vi "bt_host.vi"() -> ()   [LabVIEW 2023]
uses:
  <vilib>/Platform/TimedLoop/XDataNode/timing_clust.ctl
  <vilib>/Platform/TimedLoop/XDataNode/nitl_modes.ctl
  <vilib>/Platform/TimedLoop/XDataNode/wakeup.ctl
  <vilib>/Instr/_visa.llb/VISA Configure Serial Port (Instr).vi
  <vilib>/Platform/TimedLoop/XDataNode/XDataNode.xnode
  <vilib>/Platform/TimedLoop/XDataNode/XDNodeRunTimeDep.lvlib
panel:
  in  "탭 컨트롤 3":enum32{"Setting", "Main"}(tab)
  out "Gen ok?":bool
  out "Save_Name ok?":bool
  out "Data_Save_Name":i32[](array[numeric])
  in  "Packet Size":i32=60
  in  "설정 완료":bool
  in  "VISA resource":refnum<visa-resource-name>="COM3"
  in  "Gender":enum32{"Male", "Female"}(radio)
  in  "age":dbl
  in  "height":dbl
  out "Jitter":i32
  out "Total Data Len":i32
  out "Data":i32[](array[numeric])
  out "Received Message Count":i32
  out "Dataset":i32[](array[numeric])
  out "Adaptability(%)":sgl format="%#_3g"
  out "Batt":sgl format="%#_3g"
  in  "탭 컨트롤 2":enum32{"R/L Control", "Total Control"}(tab)
  in  "R Set":bool
  in  "R_Peak Force":i32
  in  "R_Peak":i32
  in  "R_Onset":i32
  in  "R_Release":i32
  in  "L_Release":i32
  in  "L_Onset":i32
  in  "L_Peak":i32
  in  "L_Peak Force":i32
  in  "L_Set":bool
  in  "T_Set":bool
  in  "T_Peak Force":i32
  in  "T_Peak":i32
  in  "T_Onset":i32
  in  "T_Release":i32
  in  "System Stop":bool
  in  "Stop":bool
  in  "start":bool
  out "R_GCP(%)":sgl(slide) scale=0.0..100.0
  out "L_GCP(%)":sgl(slide) scale=0.0..100.0
  in  "Control Main On/Off":bool
  out "Gait Value":cluster{"[0]":sgl, "[1]":sgl}(graph)
  out "Force":T1(graph)
  out "IMU Deg":cluster{"[0]":sgl, "[1]":sgl}(graph)
  out "COM Port":refnum<visa-resource-name>
  # "Batt(%)"
  # "Right Force Control"
  # "Left Force Control"
  # "Total Force Control"
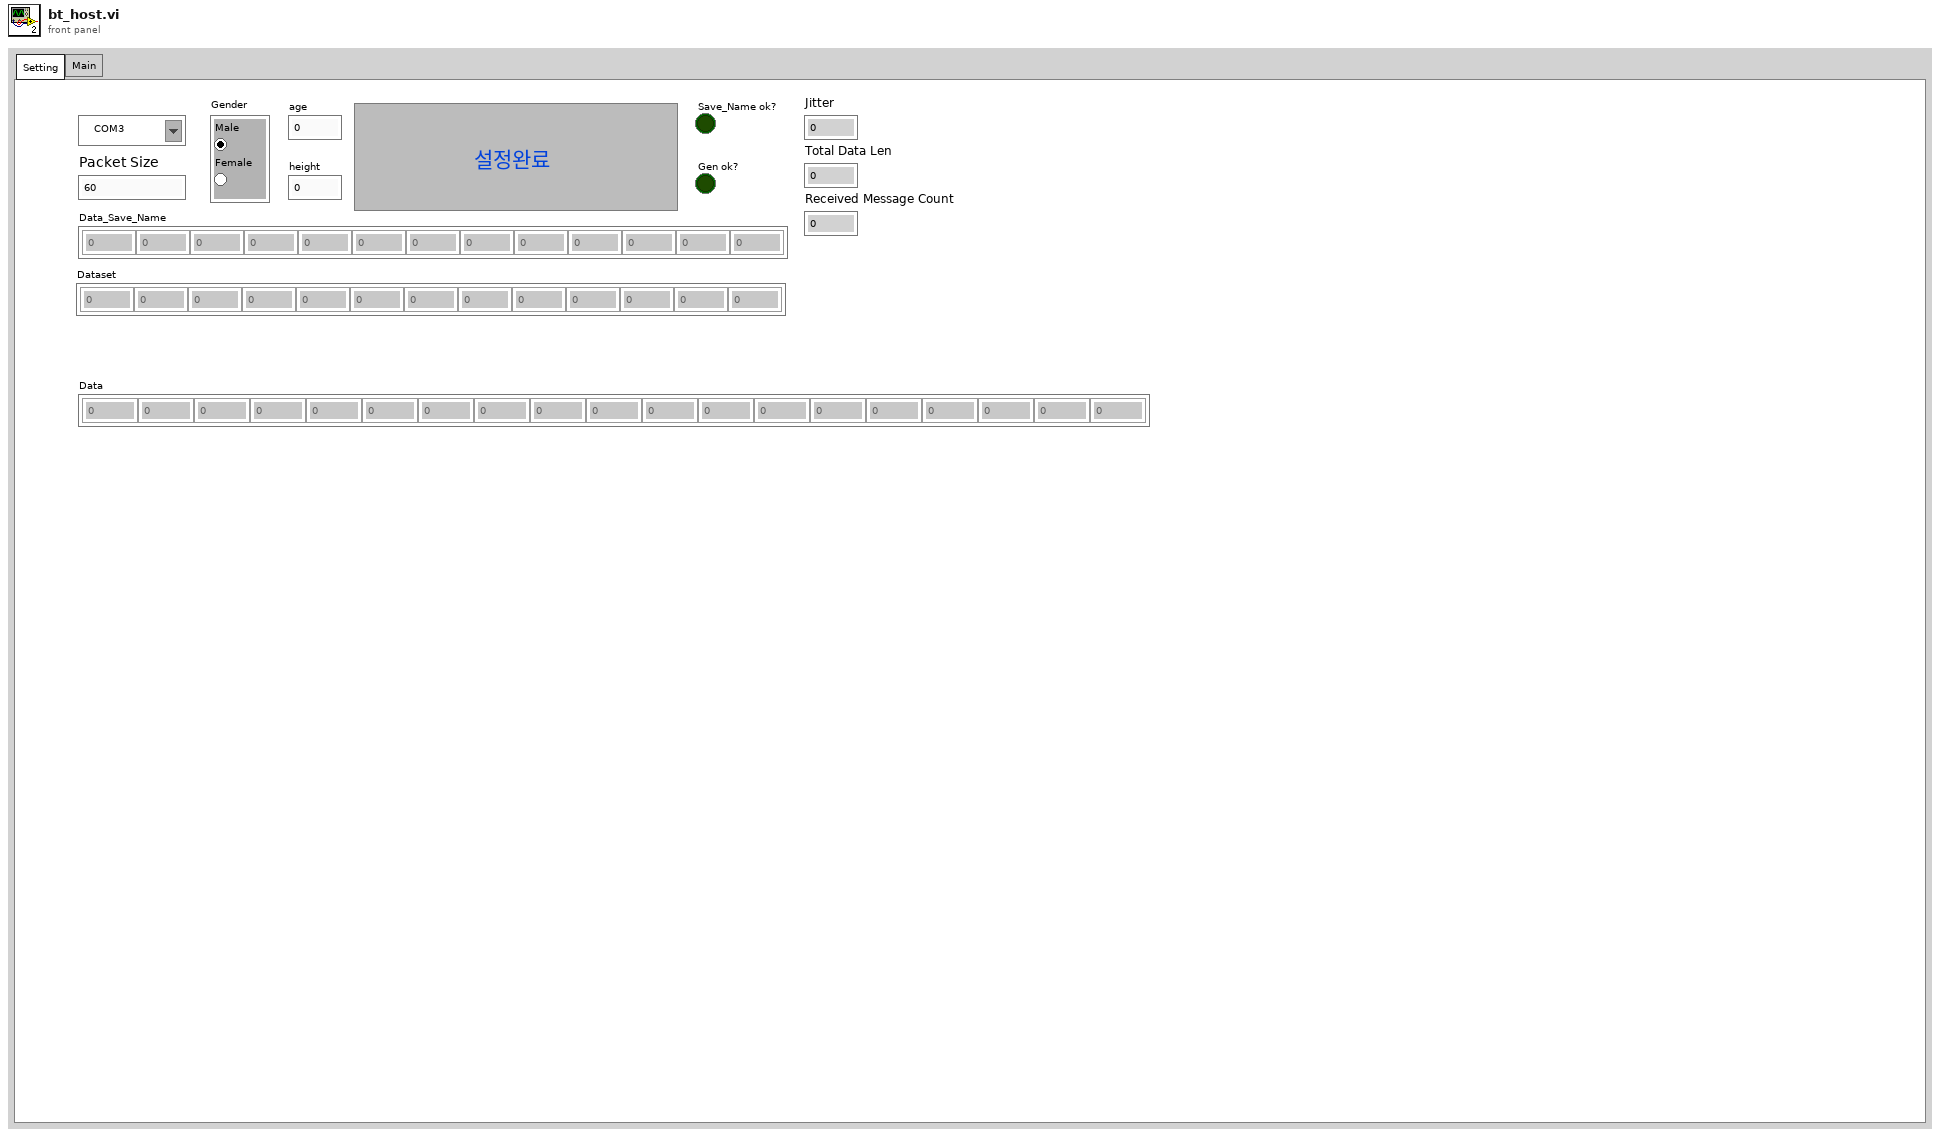
[diagram p1: front panel]
types:
  T1 = cluster{"[0]":sgl, "[1]":sgl, "[2]":sgl, "[3]":sgl}
  T2 = typedef "XDNodeRunTimeDep.lvlib/timing_clust.ctl" = cluster{"Expected End [f-1]":u64, "Actual End [f-1]":u64, "Finished Late? [f-1]":bool, "Expected End [i-1]":u64, "Actual End [i-1]":u64, "Finished Late? [i-1]":bool, "Expected Start [i]":u64, "Actual Start [i]":u64, "Expected Start [f]":u64, "Actual Start [f]":u64, "Source Name":string, "Structure Name":string, "Period":i64, "Deadline":i64, "Offset":i64, "Start":i64, "Priority":i32, "Timeout":i32, "Mode":T3, "Wakeup Reason":T4, "Error":errorcluster, "Source Type":string, "Secondary Source Type":string, "Global End Time":u64, "Global Start Time":u64, "Frame Duration":u64, "Iteration Duration":u64, "Assigned CPU":i32, "I/O Scan Engine Mode":u32}
  T3 = typedef "XDNodeRunTimeDep.lvlib/nitl_modes.ctl" = enum32{"No Change", "Process missed periods, maintain original phase", "Discard missed periods, maintain original phase", "Process missed periods, ignore original phase", "Discard missed periods, ignore original phase"}
  T4 = typedef "XDNodeRunTimeDep.lvlib/wakeup.ctl" = enum32{"Normal", "Aborted", "Asynchronous wakeup", "Timing source error", "Timed loop error", "Timeout"}
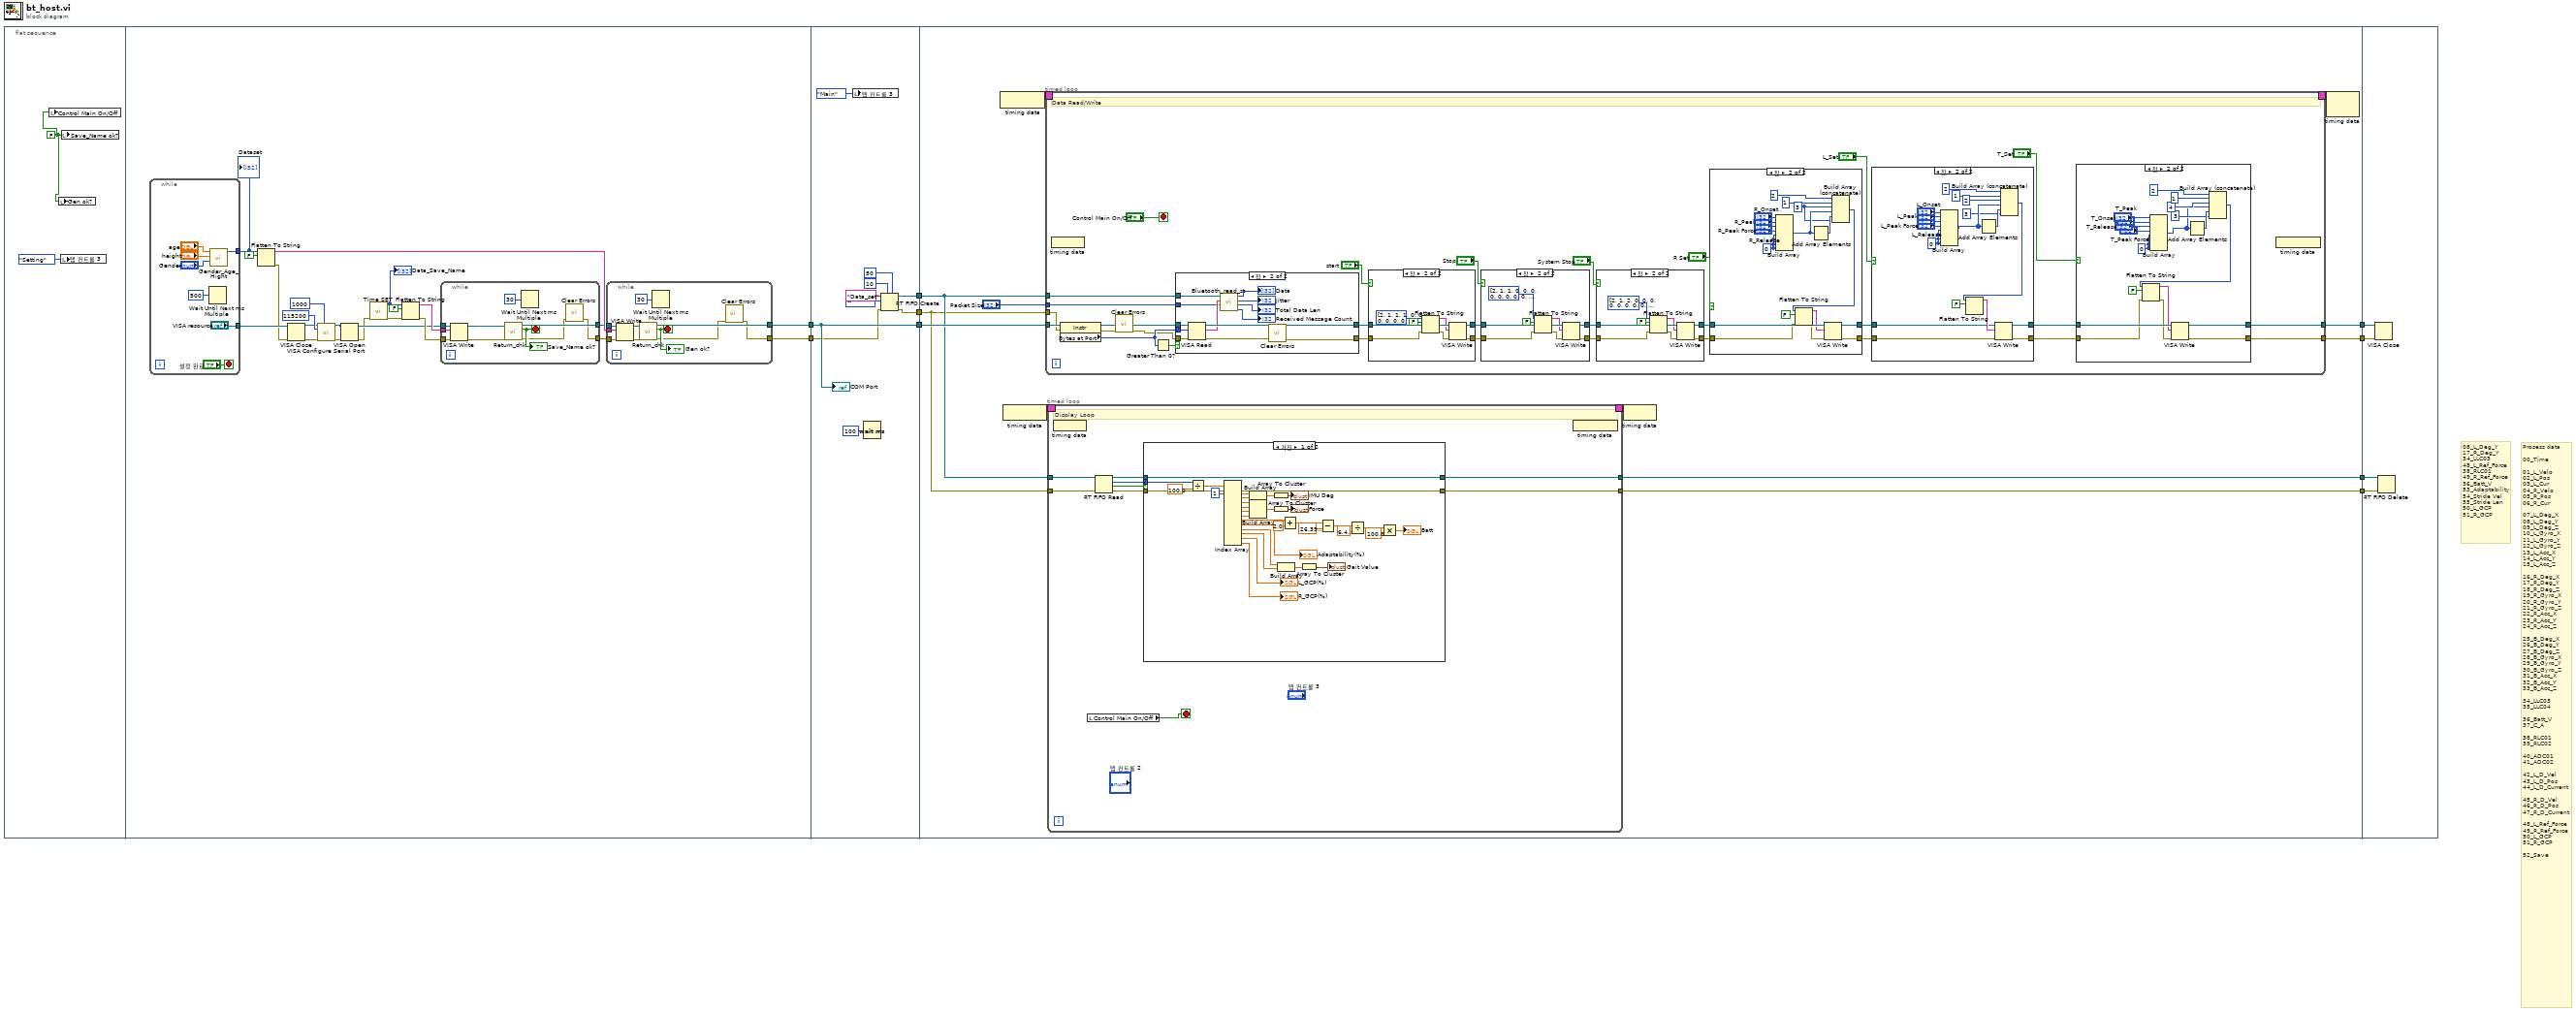
[diagram p0: block diagram]
diagram:
  # "08_L_Deg_Y\n17_R_Deg_Y\n34_LLC03\n48_L_Ref_Force\n38_RLC01\n49_R_Ref_Force\n36_Batt_V\n53_Adaptability\n54_Stride Vel\n55_Stride Len\n50_L_GCP\n51_R_GCP"
  # "Prosess data\n\n00_Time\n\n01_L_Velo\n02_L_Pos\n03_L_Cur\n04_R_Velo\n05_R_Pos\n06_R_Cur\n\n07_L_Deg_X\n08_L_Deg_Y\n09_L_Deg_Z\n10_L_Gyro_X\n11_L_Gyro_Y\n12_L_Gyro_Z\n13_L_Acc_X\n14_L_Acc_Y\n15_L_Acc_Z\n\n16_R_Deg_X\n17_R_Deg_Y\n18_R_Deg_Z\n19_R_Gyro_X\n20_R_Gyro_Y\n21_R_Gyro_Z\n22_R_Acc_X\n23_R_Acc_Y\n24_R_Acc_Z\n\n25_B_Deg_X\n26_B_Deg_Y\n27_B_Deg_Z\n28_B_Gyro_X\n29_B_Gyro_Y\n30_B_Gyro_Z\n31_B_Acc_X\n32_B_Acc_Y\n33_B_Acc_Z\n\n34_LLC03\n35_LLC04\n\n36_Batt_V\n37_C_A\n\n38_RLC01\n39_RLC02\n\n40_ADC01\n41_ADC02\n\n42_L_D_Vel\n43_L_D_Pos\n44_L_D_Current\n\n45_R_D_Vel\n46_R_D_Pos\n47_R_D_Current\n\n48_L_Ref_Force\n49_R_Ref_Force\n50_L_GCP\n51_R_GCP\n\n52_Save"
  n1 = flat-sequence {
    tunnel: [w15] -> w9
    tunnel: [w14] -> w7
    tunnel: w9 -> [w69]
    tunnel: [w69] -> w8
    tunnel: w7 -> [w66]
    tunnel: [w63] -> w6
    tunnel: [w61] -> w1
    tunnel: w8 -> [w81]
    tunnel: w6 -> [w73]
    tunnel: [w77] -> w5
    tunnel: [w76] -> w4
    tunnel: [w72] -> w3
    tunnel: [w71] -> w2
    tunnel: w1 -> [w70]
    tunnel: w5 -> [w272]
    tunnel: w4 -> [w271]
    tunnel: w3 -> [w270]
    tunnel: w2 -> [w269]
    frame #0 {
      w11 = FALSE ("Save_Name ok?")
      n2 = local write "Control Main On/Off"(w11) -> ()
      n3 = local write "Gen ok?"(w11) -> ()
      n4 = local write "탭 컨트롤 3"(enum32{"Setting", "Main"}."Setting" ("탭 컨트롤 3")) -> ()
      n5 = local write "Save_Name ok?"(w11) -> ()
    }
    frame #1 {
      n6 = while {
        tunnel: ["VISA resource"] -> w28
        tunnel: [w53] -> w18
        stop <- "설정 완료" stop-if-true
        n7 = Wait Until Next ms Multiple(millisecond multiple=u32 500 ("ms 배수")) -> ()  [unwired: 1 out]
        n8 = call "Gender_Age_Hight.vi"("Gender"="Gender", "height"="height", "age"="age") -> ("Dataset"=w53:i32[])  [unwired: 8 in]
      }
      "Dataset" <- w18
      n9 = Flatten To String(anything=w18, prepend array or string size? (T)=FALSE ("배열 또는 문자열 크기를 앞에 추가? (참)")) -> (data string=w17:string, error out=w16:errorcluster)  [unwired: 2 in, 1 out]
      n10 = VISA Close(VISA resource name=w28, error in (no error)=w16) -> (error out=w27:errorcluster)
      n11 = call-poly "VISA Configure Serial Port"("VISA resource name"=w28, "timeout (10sec)"=u32 1000, "baud rate (9600)"=u32 115200, "error in (no error)"=w27) -> ("VISA resource name out"=w30:refnum<visa-resource-name>, "error out"=w29:errorcluster)  [unwired: 10 in]
      n12 = VISA Open(error in (no error)=w29, VISA resource name=w30) -> (VISA resource name=w22:refnum<visa-resource-name>, error out=w20:errorcluster)  [unwired: 3 in]
      n13 = call "Time SET.vi"("Err_IN"=w20) -> ("Err_Out"=w21:errorcluster, "배열"=w25:i32[])  [unwired: 9 in]
      "Data_Save_Name" <- w25
      n14 = Flatten To String(anything=w25, prepend array or string size? (T)=FALSE ("배열 또는 문자열 크기를 앞에 추가? (참)"), error in (no error)=w21) -> (data string=w23:string, error out=w24:errorcluster)  [unwired: 1 in, 1 out]
      n15 = while {
        tunnel: w24 -> [w52]
        tunnel: w23 -> [w51]
        tunnel: w22 -> [w50]
        tunnel: [w43] -> w13
        tunnel: [w46] -> w12
        stop <- w47 stop-if-true
        n16 = VISA Write(VISA resource name=w50, write buffer=w51, error in (no error)=w52) -> (VISA resource name out=w49:refnum<visa-resource-name>, error out=w48:errorcluster)  [unwired: 1 out]
        n17 = call "Return_chk.vi"("에러 입력(에러 없음)"=w48, "VISA 참조 번호 입력"=w49) -> ("에러 출력"=w44:errorcluster, "불리언"=w47:bool, "VISA 참조 번호 출력"=w46:refnum<visa-resource-name>)  [unwired: 7 in]
        "Save_Name ok?" <- w47
        n18 = Wait Until Next ms Multiple(millisecond multiple=u32 30 ("ms 배수")) -> ()  [unwired: 1 out]
        n19 = call <vilib>:"Clear Errors.vi"("error in (no error)"=w44) -> ("error out"=w43:errorcluster)  [unwired: 5 in, 1 out]
      }
      n20 = while {
        tunnel: w13 -> [w42]
        tunnel: w17 -> [w41]
        tunnel: w12 -> [w40]
        tunnel: [w33] -> w14
        tunnel: [w36] -> w15
        stop <- w37 stop-if-true
        n21 = VISA Write(VISA resource name=w40, write buffer=w41, error in (no error)=w42) -> (VISA resource name out=w39:refnum<visa-resource-name>, error out=w38:errorcluster)  [unwired: 1 out]
        n22 = call "Return_chk.vi"("에러 입력(에러 없음)"=w38, "VISA 참조 번호 입력"=w39) -> ("에러 출력"=w34:errorcluster, "불리언"=w37:bool, "VISA 참조 번호 출력"=w36:refnum<visa-resource-name>)  [unwired: 7 in]
        "Gen ok?" <- w37
        n23 = Wait Until Next ms Multiple(millisecond multiple=u32 30 ("ms 배수")) -> ()  [unwired: 1 out]
        n24 = call <vilib>:"Clear Errors.vi"("error in (no error)"=w34) -> ("error out"=w33:errorcluster)  [unwired: 5 in, 1 out]
      }
    }
    frame #2 {
      n25 = local write "탭 컨트롤 3"(enum32{"Setting", "Main"}."Main" ("탭 컨트롤 3")) -> ()
      n26 = Wait (ms)(milliseconds to wait=u32 100 ("대기 시간 (ms)")) -> ()  [unwired: 1 out]
      n27 = RT FIFO Create(0:"Data_set" ("이름(이름없음)"), 1:i32[] [], 3:w66, 4:u32 10 ("크기(10)"), 6:u32 50 ("배열의 원소(1)")) -> (8:w63:refnum<k33>, 11:w61:errorcluster)  [unwired: 3 in, 1 out]
      "COM Port" <- w69
    }
    frame #3 {
      n28 = node-c288() -> (w80:T2)
      n29 = node-c288() -> (w75:T2)
      n30 = timed-loop {
        timing: w80 -> [_]
        timing-out: [_] -> w79
        tunnel: w81 -> [w158]
        tunnel: [w130] -> w76
        tunnel: [w129] -> w77
        tunnel: "Packet Size" -> [w154]
        tunnel: w73 -> [w153]
        tunnel: w70 -> [w152]
        stop <- "Control Main On/Off" stop-if-true
        # "Data Read/Write"
        n31 = node-c288() -> ()  [unwired: 1 in]
        n32 = property class="Instr"(reference=w158, error in=w152) -> (reference out=w156:refnum<visa-resource-name>, error out=w142:errorcluster, "Bytes at Port"=w155:u32)
        n33 = call <vilib>:"Clear Errors.vi"("error in (no error)"=w142) -> ("error out"=w141:errorcluster)  [unwired: 5 in, 1 out]
        n34 = Greater Than 0?(x=w155) -> (x > 0?=w157:bool)
        n35 = case shown="참" w157 {
          tunnel: w141 -> [w250 w263]
          tunnel: w156 -> [w251 w264]
          tunnel: w155 -> [_ w262]
          tunnel: [w251 w261] -> w150
          tunnel: [w250 w252] -> w149
          tunnel: w154 -> [_ w255]
          tunnel: w153 -> [_ w257]
          frame False {
          }
          frame True {
            n36 = VISA Read(VISA resource name=w264, byte count=w262, error in (no error)=w263) -> (VISA resource name out=w261:refnum<visa-resource-name>, read buffer=w256:string, error out=w253:errorcluster)  [unwired: 1 out]
            n37 = call "Bluetooth_read_st.vi"("Packet Size"=w255, "read buffer"=w256, "Data_set"=w257) -> ("Received Message Count"=→"Received Message Count":i32, "Total Data Len"=→"Total Data Len":i32, "Jitter"=→"Jitter":i32, "Data"=→"Data":i32[])  [unwired: 5 in]
            n38 = call <vilib>:"Clear Errors.vi"("error in (no error)"=w253) -> ("error out"=w252:errorcluster)  [unwired: 5 in, 1 out]
          }
        }
        n39 = case shown="참" "start" {
          tunnel: w150 -> [w241 w249]
          tunnel: w149 -> [w240 w244]
          tunnel: [w241 w248] -> w148
          tunnel: [w240 w247] -> w147
          frame False {
          }
          frame True {
            n40 = Flatten To String(anything=i32[] [2, 1, 1, 1, 0, 0, 0, 0, 0, 0, 0, 1, 3], prepend array or string size? (T)=FALSE ("배열 또는 문자열 크기를 앞에 추가? (참)"), error in (no error)=w244) -> (data string=w242:string, error out=w245:errorcluster)  [unwired: 1 in, 1 out]
            n41 = VISA Write(VISA resource name=w249, write buffer=w242, error in (no error)=w245) -> (VISA resource name out=w248:refnum<visa-resource-name>, error out=w247:errorcluster)  [unwired: 1 out]
          }
        }
        n42 = case shown="참" "Stop" {
          tunnel: w148 -> [w231 w239]
          tunnel: w147 -> [w230 w234]
          tunnel: [w231 w238] -> w145
          tunnel: [w230 w237] -> w144
          frame False {
          }
          frame True {
            n43 = Flatten To String(anything=i32[] [2, 1, 1, 0, 0, 0, 0, 0, 0, 0, 0, 0, 3], prepend array or string size? (T)=FALSE ("배열 또는 문자열 크기를 앞에 추가? (참)"), error in (no error)=w234) -> (data string=w233:string, error out=w235:errorcluster)  [unwired: 1 in, 1 out]
            n44 = VISA Write(VISA resource name=w239, write buffer=w233, error in (no error)=w235) -> (VISA resource name out=w238:refnum<visa-resource-name>, error out=w237:errorcluster)  [unwired: 1 out]
          }
        }
        n45 = case shown="참" "System Stop" {
          tunnel: w145 -> [w221 w229]
          tunnel: w144 -> [w220 w224]
          tunnel: [w221 w228] -> w140
          tunnel: [w220 w227] -> w139
          frame False {
          }
          frame True {
            n46 = Flatten To String(anything=i32[] [2, 1, 2, 0, 0, 0, 0, 0, 0, 0, 0, 2, 3], prepend array or string size? (T)=FALSE ("배열 또는 문자열 크기를 앞에 추가? (참)"), error in (no error)=w224) -> (data string=w223:string, error out=w225:errorcluster)  [unwired: 1 in, 1 out]
            n47 = VISA Write(VISA resource name=w229, write buffer=w223, error in (no error)=w225) -> (VISA resource name out=w228:refnum<visa-resource-name>, error out=w227:errorcluster)  [unwired: 1 out]
          }
        }
        n48 = case shown="참" "R Set" {
          tunnel: w140 -> [w201 w217]
          tunnel: w139 -> [w200 w214]
          tunnel: [w201 w219] -> w135
          tunnel: [w200 w218] -> w134
          frame False {
          }
          frame True {
            w206 = 0 ("원소")
            w203 = 3 ("원소")
            n49 = Build Array("R_Onset", "R_Peak", "R_Release", "R_Peak Force", w206, w206, w206, w206) -> (w205:i32[])
            n50 = Add Array Elements(numeric array=w205) -> (sum=w204:i32)
            n51 = Build Array (concatenate)(2 ("원소"), 1 ("원소"), w203, w205, w204, w203) -> (w202:i32[])
            n52 = Flatten To String(anything=w202, prepend array or string size? (T)=FALSE ("배열 또는 문자열 크기를 앞에 추가? (참)"), error in (no error)=w214) -> (data string=w216:string, error out=w215:errorcluster)  [unwired: 1 in, 1 out]
            n53 = VISA Write(VISA resource name=w217, write buffer=w216, error in (no error)=w215) -> (VISA resource name out=w219:refnum<visa-resource-name>, error out=w218:errorcluster)  [unwired: 1 out]
          }
        }
        n54 = case shown="참" "L_Set" {
          tunnel: w135 -> [w181 w193]
          tunnel: w134 -> [w180 w192]
          tunnel: [w180 w191] -> w132
          tunnel: [w181 w190] -> w133
          frame False {
          }
          frame True {
            w182 = 0 ("원소")
            n55 = Build Array("L_Onset", "L_Peak", "L_Release", "L_Peak Force", w182, w182, w182, w182) -> (w185:i32[])
            n56 = Add Array Elements(numeric array=w185) -> (sum=w187:i32)
            n57 = Build Array (concatenate)(2 ("원소"), 1 ("원소"), 2 ("원소"), w185, w187, 3 ("원소")) -> (w183:i32[])
            n58 = Flatten To String(anything=w183, prepend array or string size? (T)=FALSE ("배열 또는 문자열 크기를 앞에 추가? (참)")) -> (data string=w195:string)  [unwired: 2 in, 2 out]
            n59 = VISA Write(VISA resource name=w193, write buffer=w195, error in (no error)=w192) -> (VISA resource name out=w190:refnum<visa-resource-name>, error out=w191:errorcluster)  [unwired: 1 out]
          }
        }
        n60 = case shown="참" "T_Set" {
          tunnel: w133 -> [w160 w177]
          tunnel: w132 -> [w159 w174]
          tunnel: [w160 w179] -> w130
          tunnel: [w159 w178] -> w129
          frame False {
          }
          frame True {
            w172 = 0 ("원소")
            n61 = Build Array("T_Onset", "T_Peak", "T_Release", "T_Peak Force", w172, w172, w172, w172) -> (w162:i32[])
            n62 = Add Array Elements(numeric array=w162) -> (sum=w165:i32)
            n63 = Build Array (concatenate)(2 ("원소"), 1 ("원소"), 4 ("원소"), w162, w165, 3 ("원소")) -> (w161:i32[])
            n64 = Flatten To String(anything=w161, prepend array or string size? (T)=FALSE ("배열 또는 문자열 크기를 앞에 추가? (참)"), error in (no error)=w174) -> (data string=w175:string, error out=w176:errorcluster)  [unwired: 1 in, 1 out]
            n65 = VISA Write(VISA resource name=w177, write buffer=w175, error in (no error)=w176) -> (VISA resource name out=w179:refnum<visa-resource-name>, error out=w178:errorcluster)  [unwired: 1 out]
          }
        }
        n66 = node-c288() -> ()  [unwired: 1 out]
      }
      n67 = timed-loop {
        timing: w75 -> [_]
        timing-out: [_] -> w74
        tunnel: w73 -> [w90]
        tunnel: [w85] -> w71
        tunnel: [w84] -> w72
        tunnel: w70 -> [w82]
        stop <- w83 stop-if-true
        # "Display Loop"
        n68 = node-c288() -> ()  [unwired: 1 in]
        n69 = local read "Control Main On/Off"() -> (w83:bool)
        n70 = RT FIFO Read(0:w90, 3:w82) -> (8:w86:refnum<k33>, 9:w88:i32[], 10:w89:bool, 11:w87:errorcluster)  [unwired: 2 in, 1 out]
        n71 = case shown="거짓" w89 {
          tunnel: w88 -> [w119 _]
          tunnel: w87 -> [w121 w124]
          tunnel: w86 -> [w122 w123]
          tunnel: [w121 w124] -> w85
          tunnel: [w122 w123] -> w84
          frame False {
            n72 = Divide(x=w119, y=sgl 100.0) -> (x/y=w118:sgl[])
            n73 = Index Array(array=w118, index #1=1 ("인덱스")) -> (element #1=w116:sgl, element #2=w115:sgl, element #3=w112:sgl, element #4=w111:sgl, element #5=w110:sgl, element #6=w109:sgl, element #7=w100:sgl, element #8=→"Adaptability(%)":sgl, element #9=w94:sgl, element #10=w91:sgl, element #11=→"L_GCP(%)":sgl, element #12=→"R_GCP(%)":sgl)  [unwired: 11 in]
            n74 = Build Array(w116, w115) -> (w114:sgl[])
            n75 = Build Array(w112, w111, w110, w109) -> (w108:sgl[])
            n76 = Array To Cluster(array=w114) -> (cluster=→"IMU Deg":cluster{"[0]":sgl, "[1]":sgl})
            n77 = Array To Cluster(array=w108) -> (cluster=→"Force":T1)
            n78 = Build Array(w94, w91) -> (w97:sgl[])
            n79 = Add(x=w100, y=sgl 2.0) -> (x+y=w98:sgl)
            n80 = Array To Cluster(array=w97) -> (cluster=→"Gait Value":cluster{"[0]":sgl, "[1]":sgl})
            n81 = Subtract(x=w98, y=sgl 26.4 ("x")) -> (x-y=w106:sgl)
            n82 = Divide(x=w106, y=sgl 6.4) -> (x/y=w104:sgl)
            n83 = Multiply(x=w104, y=sgl 100.0) -> (x*y=→"Batt":sgl)
          }
          frame True {
          }
        }
        n84 = node-c288() -> ()  [unwired: 1 out]
      }
      n85 = node-c288(w74) -> ()
      n86 = node-c288(w79) -> ()  [unwired: 1 out]
    }
    frame #4 {
      n87 = VISA Close(VISA resource name=w271, error in (no error)=w272) -> ()  [unwired: 1 out]
      n88 = RT FIFO Delete(0:w270, 3:w269) -> ()  [unwired: 1 in, 1 out]
    }
  }
